vi "TestFindFaces_cmd.vi"() -> ()   [LabVIEW 2018]
uses:
  <vilib>/Utility/sysdir.llb/System Directory Type.ctl
  <vilib>/ptbypt/NI_PtbyPt.lvlib
panel:
  out "Mean Execution Time (s)":dbl
  in  "stop":bool
  out "Execution Time":dbl(graph)
  out "image with faces":picture
  # "This VI Demonstrates using the System Exec VI to call Python with OpenCV to do simple facial recognition on an image and benchmarks its execution time for comparison with other methods of communicating with Python in LabVIEW. \nIt will read an image file and draw a box around the face."
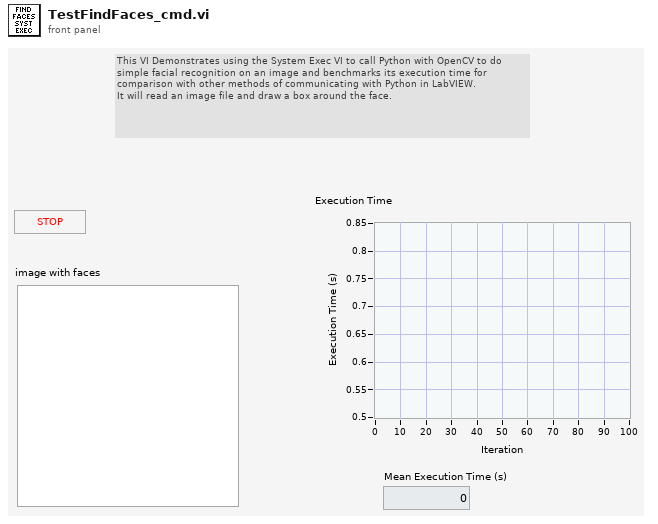
[diagram p1: front panel]
types:
  T1 = typedef "System Directory Type.ctl" = i32
  T2 = typedef "imagedata.ctl" = cluster{"image type":i32, "image depth":i32, "image":u8[], "mask":u8[], "colors":u32[], "Rectangle":cluster{"left":i16, "top":i16, "right":i16, "bottom":i16}}
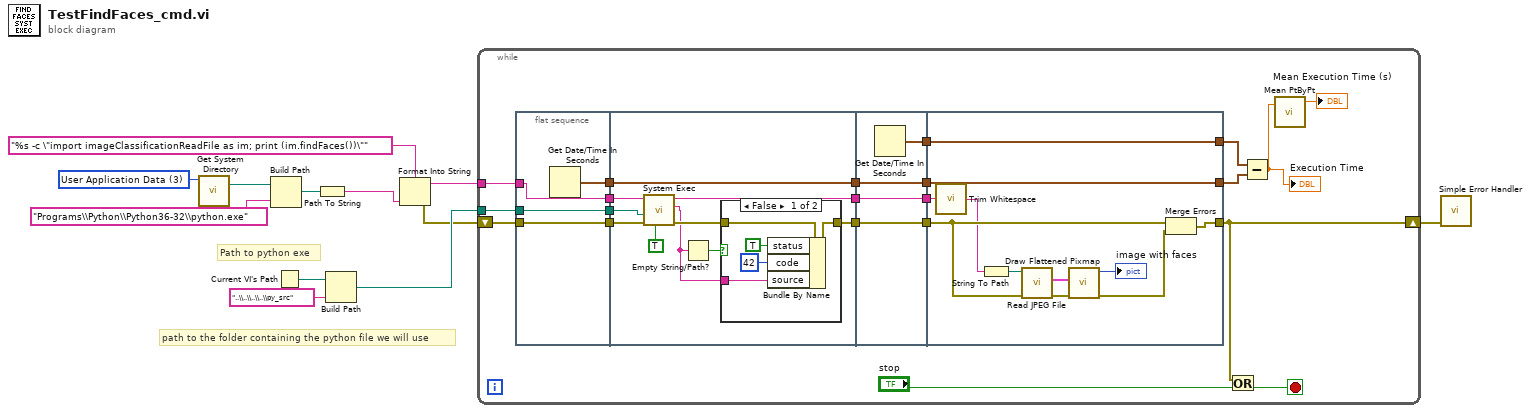
[diagram p0: block diagram]
diagram:
  w11 = T1 3 items=["User Home"=0, "User Desktop"=1, "User Documents"=2, "User Application Data"=3, "User Preferences"=4, "User Temporary"=5, "Public Documents"=6, "Public Application Data"=7, "Public Preferences"=8, "Public Cache"=13, "System Core Libraries"=9, "System Installed Libraries"=10, "Application Files"=11, "Boot Volume Root"=12] ("system directory type")
  # "Path to python exe"
  # "path to the folder containing the python file we will use"
  n1 = call <vilib>:"Get System Directory.vi"("system directory type"=w11) -> ("system directory"=w8:path)  [unwired: 10 in]
  n2 = Build Path(base path=w8, name or relative path="Programs\\Python\\Python36-32\\python.exe") -> (appended path=w6:path)
  n3 = Current VI's Path() -> (path=w10:path)
  n4 = Path To String(path=w6) -> (string=w4:string)
  n5 = Build Path(base path=w10, name or relative path="..\\..\\..\\..\\py_src") -> (appended path=w2:path)
  n6 = Format Into String(format string="%s -c \"import imageClassificationReadFile as im; print (im.findFaces())\"", w4) -> (resulting string=w3:string, error out=w1:errorcluster)  [unwired: 2 in]
  n7 = while {
    shift-right: [w27] -> w12
    shift-left: w1 -> [w33]
    tunnel: w3 -> [w17]
    tunnel: w2 -> [w16]
    stop <- w28 stop-if-true
    n8 = flat-sequence {
      tunnel: w16 -> [w36]
      tunnel: w33 -> [w37]
      tunnel: [w37] -> w22
      tunnel: [w36] -> w21
      tunnel: [w35] -> w19
      tunnel: [w34] -> w18
      tunnel: w17 -> [w34]
      tunnel: [w40] -> w32
      tunnel: [w44] -> w31
      tunnel: w22 -> [w45]
      tunnel: w21 -> [w38]
      tunnel: [w47] -> w20
      tunnel: w19 -> [w47]
      tunnel: w18 -> [w43]
      tunnel: w32 -> [w57]
      tunnel: w31 -> [w56]
      tunnel: [w57] -> w26
      tunnel: [w56] -> w25
      tunnel: [w55] -> w24
      tunnel: [w54] -> w23
      tunnel: w20 -> [w54]
      tunnel: [w66] -> w29
      tunnel: [w67] -> w30
      tunnel: [w61] -> w27
      tunnel: w26 -> [w62]
      tunnel: w25 -> [w63]
      tunnel: w24 -> [w67]
      tunnel: w23 -> [w66]
      frame #0 {
        n9 = Get Date/Time In Seconds() -> (seconds since 1Jan1904=w35:timestamp)
      }
      frame #1 {
        n10 = call <vilib>:"System Exec.vi"("run minimized? (F)"=TRUE, "error in (no error)"=w45, "working directory"=w38, "command line"=w43) -> ("error out"=w41:errorcluster, "standard error"=w39:string, "standard output"=w44:string)  [unwired: 4 in, 1 out]
        n11 = Empty String/Path?(string/path=w39) -> (empty?=w42:bool)
        n12 = case shown="False" w42 {
          tunnel: w41 -> [w52 w53]
          tunnel: [w48 w53] -> w40
          tunnel: w39 -> [w50 _]
          frame False {
            n13 = Bundle By Name(cluster=w52, "status"=TRUE, "code"=42, "source"=w50) -> (w48:errorcluster)
          }
          frame True {
          }
        }
      }
      frame #2 {
        n14 = Get Date/Time In Seconds() -> (seconds since 1Jan1904=w55:timestamp)
      }
      frame #3 {
        n15 = call <vilib>:"Trim Whitespace.vi"("string"=w63) -> ("trimmed string"=w59:string)  [unwired: 1 in]
        n16 = String To Path(string=w59) -> (path=w65:path)
        n17 = call <vilib>:"Read JPEG File.vi"("error in (no error)"=w62, "path to JPEG file"=w65) -> ("error out"=w60:errorcluster, "image data"=w64:T2)  [unwired: 7 in, 1 out]
        n18 = call <vilib>:"Draw Flattened Pixmap.vi"("image data"=w64) -> ("new picture"=→"image with faces":picture)  [unwired: 8 in]
        n19 = Merge Errors(w62, w60) -> (w61:errorcluster)
      }
    }
    n20 = Or(x=w27, y="stop") -> (x .or. y?=w28:bool)
    n21 = Subtract(x=w30, y=w29) -> (x-y=w15:dbl)
    "Execution Time" <- w15
    n22 = call <vilib>:"Mean PtByPt.vi"("x"=w15) -> ("mean"=→"Mean Execution Time (s)":dbl)  [unwired: 3 in, 1 out]
  }
  n23 = call <vilib>:"Simple Error Handler.vi"("error in (no error)"=w12) -> ()  [unwired: 4 in, 5 out]
